vi "CRYAdd Steps.vi"() -> ()   [LabVIEW 2013]
doc: "This Example will search through the selected directory for specified files, populate the Tree control with the directory hierarchy, and then close the folder glyphs.\n This VI also demonestrates the use of the ActiveItem:RowNumber property that displays the active items row number. You could select the row number of the\n item to display its tag and cell string as well. Go to File >> VI Properties >> Documentation or Right click on the VI icon and select VI Properties. The\ncontext help window (Ctrl-h) will display detailed description of controls and indicators when you hover over them. \nInstructions:\n1. Specify the directory and the pattern to search for (i.e *.txt).\n2. Run the VI.\n3. Click on any item on the tree to display its tag and string."
uses:
  <vilib>/event_ctls.llb/eventvkey.ctl
  CRYProject/CRYProject Editor Global.vi
  CRYStepSetup/CRYStepSetup Global.vi
  CRYWindow/SubVI/CRYMain Sub Window Global.vi
  CRYMainGlobal.vi
  CRYCurveLibrary/Global/CRYCurve Library Global.vi
panel:
  in  "Option":bool
  in  "Remove":bool
  in  "StateOut":bool
  in  "Refresh":bool
  in  "UpdateAddStep":bool
  in  "stop":bool
  in  "Board Tab":enum32{"Step", "Sequence"}(tab)
  in  "Steps":string(tree)
  in  "Sequences":string(tree)
  in  "Item Remove":bool
  in  "AllChange":bool
  out "Help":string
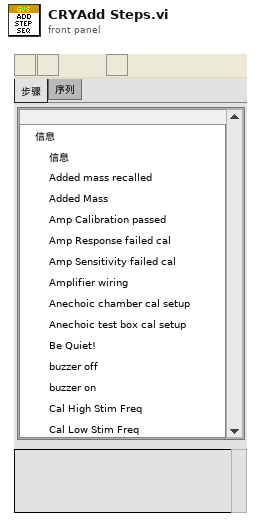
[diagram p1: front panel]
types:
  T1 = cluster{"Content":string, "Name":string, "Level":u32, "Category":string}[]
  T2 = enum16{"OK", "Yes", "YesNo", "YesNoCancel", "ReplaceAppend"}
  T3 = typedef "eventvkey.ctl" = enum16{"ASCII", "Enter", "Return", "Shift", "Ctrl", "Alt", "Cmd", "Opt", "Caps", "NumLock", "Clear", "Break", "Up", "Down", "Left", "Right", "Insert", "Delete", "Home", "End", "PageUp", "PageDown", "Escape", "Help", "Pause", "ScrollLock", "F1", "F2", "F3", "F4", "F5", "F6", "F7", "F8", "F9", "F10", "F11", "F12", "F13", "F14", "F15", "F16", "F17", "F18", "F19", "F20", "F21", "F22", "F23", "F24", "Play", "VolumeUp", "VolumeDown", "Mute", "Two Byte Char"}
  T4 = enum32{"Invalid", "Standard", "Closed", "Hidden", "Minimized", "Maximized"}
  T5 = typedef "LVPoint32TypeDef.ctl" = cluster{"Horizontal":i32, "Vertical":i32}
  T6 = cluster{"Content":string, "Name":string, "Level":u32, "Category":string}
  T7 = typedef "CRYCurveLib Info Cluster.ctl" = cluster{"GroupingState":string}
  T8 = typedef "LVRectTypeDef.ctl" = cluster{"Left":i16, "Top":i16, "Right":i16, "Bottom":i16}
  T9 = cluster{"EventName":string, "Arg1":string, "Arg1 2":string, "Numeric":dbl, "Arg1 3":string}
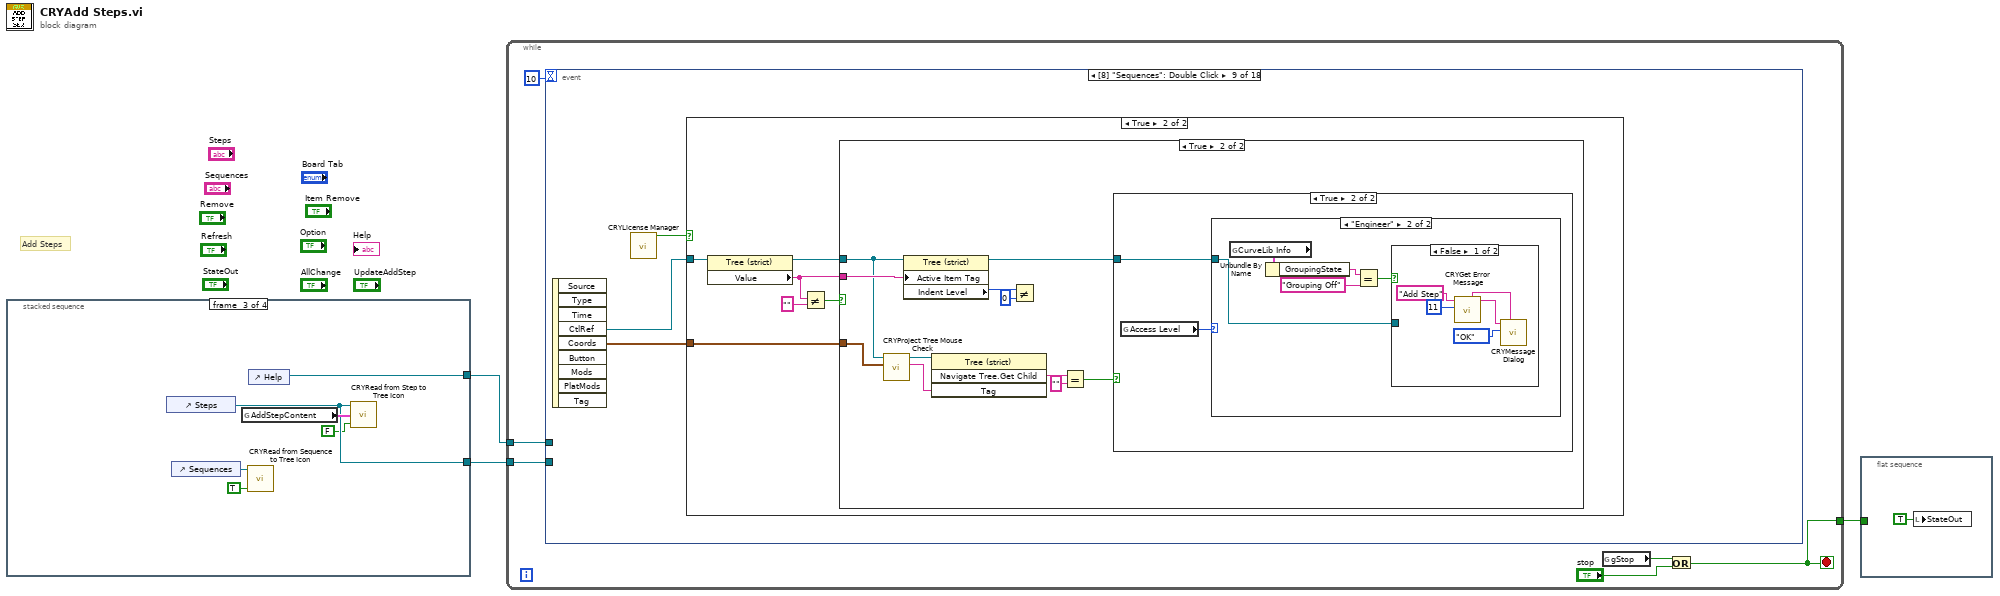
[diagram p0: block diagram]
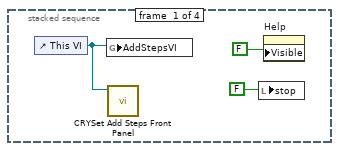
[diagram p2: hidden frame]
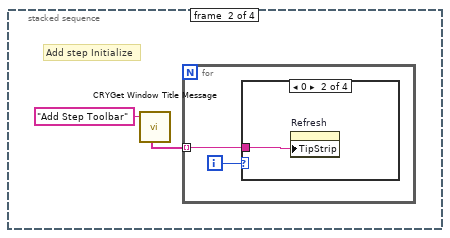
[diagram p3: hidden frame]
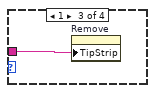
[diagram p5: hidden frame]
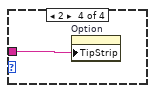
[diagram p6: hidden frame]
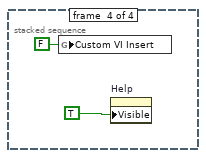
[diagram p7: hidden frame]
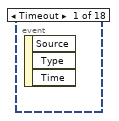
[diagram p8: hidden frame]
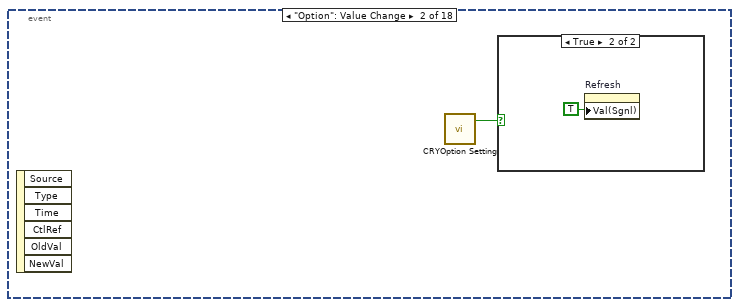
[diagram p9: hidden frame]
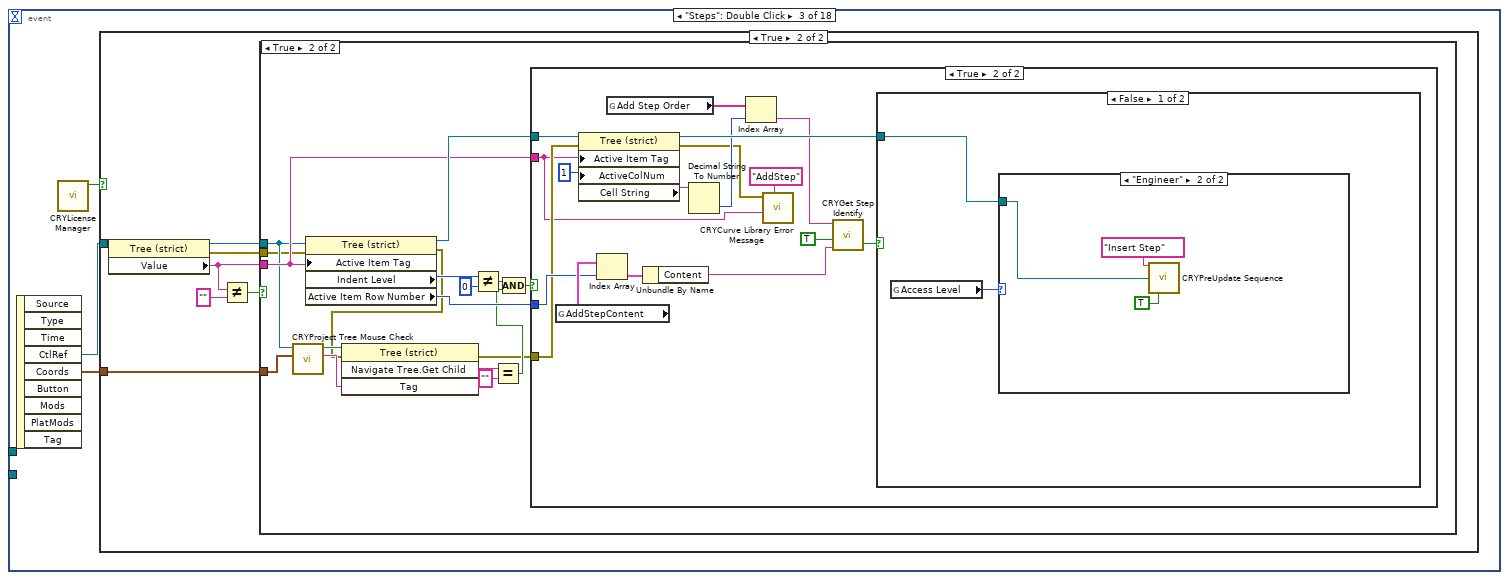
[diagram p11: hidden frame]
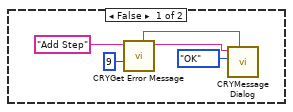
[diagram p12: hidden frame]
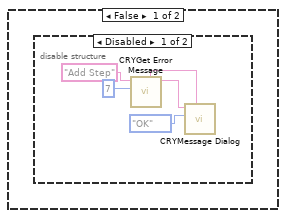
[diagram p13: hidden frame]
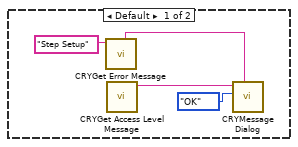
[diagram p16: hidden frame]
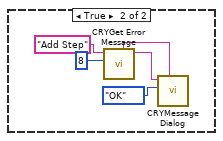
[diagram p17: hidden frame]
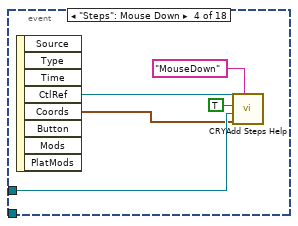
[diagram p18: hidden frame]
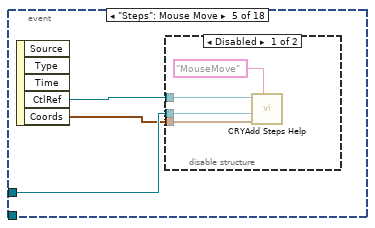
[diagram p19: hidden frame]
diagram:
  # "Add Steps"
  n1 = stacked-sequence {
    tunnel: [_ _ w19 _] -> w3
    tunnel: [_ _ w17 _] -> w2
    frame #0 {
      n2 = control-ref of="This VI"() -> (w4:refnum<vi>)
      n3 = global write "CRYProject Editor Global.vi" "AddStepsVI"(w4) -> ()
      n4 = call "CRYSet Add Steps Front Panel.vi"("Vi Ref"=w4) -> ()  [unwired: 11 in]
      n5 = local write "stop"(FALSE ("stop")) -> ()
      n6 = property on="Help" class="Str"("Visible"=FALSE) -> ()  [unwired: 2 in, 2 out]
    }
    frame #1 {
      # "Add step Initialize"
      n7 = call "CRYGet Window Title Message.vi"("Kind"="Add Step Toolbar") -> ("Tip Strip"=w8:string[])  [unwired: 5 in, 5 out]
      n8 = for {
        tunnel: w8 -> [w9] mode=indexing
        i -> [w10]
        n9 = case shown="0" w10 {
          tunnel: w9 -> [_ w11 w12 w13]
          frame Default {
          }
          frame 0 {
            n10 = property on="Refresh" class="Bool (strict)"("TipStrip"=w11) -> ()  [unwired: 2 in, 2 out]
          }
          frame 1 {
            n11 = property on="Remove" class="Bool (strict)"("TipStrip"=w12) -> ()  [unwired: 2 in, 2 out]
          }
          frame 2 {
            n12 = property on="Option" class="Bool (strict)"("TipStrip"=w13) -> ()  [unwired: 2 in, 2 out]
          }
        }
      }
    }
    frame #2 {
      n13 = control-ref of="Steps"() -> (w17:refnum<vi>)
      n14 = control-ref of="Sequences"() -> (w15:refnum<vi>)
      n15 = global read "CRYProject Editor Global.vi" "AddStepContent"() -> (w18:T1)
      n16 = call "CRYRead from Sequence to Tree Icon.vi"("Is Refresh?"=TRUE, "StepsRef in"=w15) -> ()  [unwired: 8 in, 2 out]
      n17 = control-ref of="Help"() -> (w19:refnum<vi>)
      n18 = call "CRYRead from Step to Tree Icon.vi"("Is Refresh?"=FALSE ("Type In"), "StepContentIn"=w18, "StepsRef in"=w17) -> ()  [unwired: 3 out]
    }
    frame #3 {
      n19 = global write "CRYStepSetup Global.vi" "Custom VI Insert"(FALSE ("Custom VI Insert")) -> ()
      n20 = property on="Help" class="Str"("Visible"=TRUE) -> ()  [unwired: 2 in, 2 out]
    }
  }
  n21 = while {
    tunnel: w3 -> [w26]
    tunnel: w2 -> [w25]
    tunnel: [w22] -> w1
    stop <- w22 stop-if-true
    n22 = event shown="[8] \"Sequences\": Double Click" {
      selector: _ -> [_ _ _ _ _ _ _ _ _ _ _ _ _ _ _ _ _ _]
      dyn-events: _ -> [_ _ _ _ _ _ _ _ _ _ _ _ _ _ _ _ _ _]
      timeout: 10 -> [_ _ _ _ _ _ _ _ _ _ _ _ _ _ _ _ _ _]
      tunnel: w26 -> [_ _ _ w101 w104 w113 _ _ _ _ _ _ _ _ _ _ _ _]
      tunnel: w25 -> [_ _ _ _ _ _ _ _ _ _ _ _ _ _ _ _ _ w260]
      event Timeout {
        n23 = event-data() -> ()  [unwired: 4 out]
      }
      event "Option": Value Change {
        n24 = event-data() -> ()  [unwired: 7 out]
        n25 = call "CRYOption Setting.vi"() -> ("OK Flag"=w28:bool)  [unwired: 9 in, 2 out]
        n26 = case shown="True" w28 {
          frame False {
          }
          frame True {
            n27 = property on="Refresh" class="Bool (strict)"("Val(Sgnl)"=TRUE ("Value (Signaling)")) -> ()  [unwired: 2 in, 2 out]
          }
        }
      }
      event "Steps": Double Click {
        n28 = event-data() -> ("CtlRef"=w32:refnum<vi>, "Coords"=w31:T5)  [unwired: 8 out]
        n29 = call "CRYLicense Manager.vi"() -> ("Test Result"=w30:bool)  [unwired: 10 in, 1 out]
        n30 = case shown="True" w30 {
          tunnel: w32 -> [_ w44]
          tunnel: w31 -> [_ w39]
          frame False {
            n31 = call "CRYGet Error Message.vi"("Error No"=9, "Kind"="Add Step") -> ("Message"=w33:string, "Window Title"=w37:string)  [unwired: 4 in, 4 out]
            n32 = call "CRYMessage Dialog.vi"("Window Title"=w37, "YesNoCancel"=T2."OK", "Message Content"=w33) -> ()  [unwired: 7 in, 2 out]
          }
          frame True {
            n33 = property class="Tree (strict)"(reference=w44) -> (reference out=w43:refnum<vi>, error out=w38:errorcluster, "Value"=w42:string)  [unwired: 1 in]
            n34 = Not Equal?(x=w42, y="") -> (x != y?=w40:bool)
            n35 = case shown="True" w40 {
              tunnel: w43 -> [_ w56]
              tunnel: w42 -> [_ w61]
              tunnel: w39 -> [_ w55]
              tunnel: w38 -> [_ w52]
              frame False {
                n36 = disable-structure shown="Disabled" {
                  frame Disabled {
                    n37 = call "CRYGet Error Message.vi"("Error No"=7, "Kind"="Add Step") -> ("Message"=w48:string, "Window Title"=w47:string)  [unwired: 4 in, 4 out]
                    n38 = call "CRYMessage Dialog.vi"("Window Title"=w47, "YesNoCancel"=T2."OK", "Message Content"=w48) -> ()  [unwired: 7 in, 2 out]
                  }
                  frame Enabled {
                  }
                }
              }
              frame True {
                n39 = call "CRYProject Tree Mouse Check.vi"("Coords In"=w55, "Tree Reference In"=w56) -> ("Clicked String Out"=w57:string, "Tree Reference Out"=w58:refnum<vi>)  [unwired: 8 in]
                n40 = property class="Tree (strict)"(reference=w56, error in=w52, "Active Item Tag"=w61) -> (reference out=w66:refnum<vi>, error out=w51:errorcluster, "Indent Level"=w65:i32, "Active Item Row Number"=w64:i32)
                n41 = invoke class="Tree (strict)" method="Navigate Tree.Get Child"(reference=w58, error in=w51, "Tag"=w57) -> (error out=w50:errorcluster, "Navigate Tree:Get Child"=w59:string)  [unwired: 1 in, 2 out]
                n42 = Not Equal?(x=w65, y=0) -> (x != y?=w62:bool)
                n43 = Equal?(x=w59, y="") -> (x = y?=w53:bool)
                n44 = Compound Arithmetic op=AND(w62, w53) -> (w54:bool)
                n45 = case shown="True" w54 {
                  tunnel: w64 -> [_ w78]
                  tunnel: w61 -> [_ w67]
                  tunnel: w66 -> [_ w77]
                  tunnel: w50 -> [_ w70]
                  frame False {
                  }
                  frame True {
                    n46 = global read "CRYProject Editor Global.vi" "AddStepContent"() -> (w80:T1)
                    n47 = property class="Tree (strict)"(reference=w77, error in=w70, "Active Item Tag"=w67, "ActiveColNum"=1 ("Active Cell:Active Column Number")) -> (reference out=w74:refnum<vi>, error out=w69:errorcluster, "Cell String"=w75:string)
                    n48 = Index Array(array=w80, index=w78) -> (element=w81:T6)
                    n49 = global read "CRYMainGlobal.vi" "Add Step Order"() -> (w73:string[])
                    n50 = Unbundle By Name(w81) -> ("Content"=w82:string)
                    n51 = Decimal String To Number(string=w75) -> (number=w72:i32)  [unwired: 2 in, 1 out]
                    n52 = Index Array(array=w73, index=w72) -> (element=w71:string)
                    n53 = call "CRYCurve Library Error Message.vi"("sAction"="AddStep", "sData"=w67, "error IO"=w69) -> ()  [unwired: 9 in]
                    n54 = call "CRYGet Step Identify.vi"("Unflatten Seq-step setup"=w82, "Help?"=TRUE, "Category Name In"=w71) -> ("Error?"=w79:bool)  [unwired: 1 in, 7 out]
                    n55 = case shown="False" w79 {
                      tunnel: w74 -> [w84 _]
                      frame False {
                        n56 = global read "CRYMainGlobal.vi" "Access Level"() -> (w85:enum16{"Engineer", "Technician", "Operator"})
                        n57 = case shown="\"Engineer\"" w85 {
                          tunnel: w84 -> [_ w92]
                          frame Default {
                            n58 = call "CRYGet Error Message.vi"("Kind"="Step Setup") -> ("Window Title"=w87:string)  [unwired: 5 in, 5 out]
                            n59 = call "CRYGet Access Level Message.vi"() -> ("Multibyte string"=w89:string)  [unwired: 11 in]
                            n60 = call "CRYMessage Dialog.vi"("Window Title"=w87, "YesNoCancel"=T2."OK", "Message Content"=w89) -> ()  [unwired: 7 in, 2 out]
                          }
                          frame "Engineer" {
                            n61 = call "CRYPreUpdate Sequence.vi"("EventName"="Insert Step" ("Name"), "AddSteps"=w92, "AllChangeFlg"=TRUE) -> ()  [unwired: 13 in]
                          }
                        }
                      }
                      frame True {
                        n62 = call "CRYGet Error Message.vi"("Error No"=8, "Kind"="Add Step") -> ("Message"=w96:string, "Window Title"=w95:string)  [unwired: 4 in, 4 out]
                        n63 = call "CRYMessage Dialog.vi"("Window Title"=w95, "YesNoCancel"=T2."OK", "Message Content"=w96) -> ()  [unwired: 7 in, 2 out]
                      }
                    }
                  }
                }
              }
            }
          }
        }
      }
      event "Steps": Mouse Down {
        n64 = event-data() -> ("CtlRef"=w102:refnum<vi>, "Coords"=w100:T5)  [unwired: 7 out]
        n65 = call "CRYAdd Steps Help.vi"("Option"="MouseDown", "Coords"=w100, "Help"=w101, "Help?"=TRUE, "AddSteps"=w102) -> ()  [unwired: 7 out]
      }
      event "Steps": Mouse Move {
        n66 = event-data() -> ("CtlRef"=w105:refnum<vi>, "Coords"=w103:T5)  [unwired: 4 out]
        n67 = disable-structure shown="Disabled" {
          disable-tunnel: w105 -> [w109 _]
          disable-tunnel: w104 -> [w108 _]
          disable-tunnel: w103 -> [w107 _]
          frame Disabled {
            n68 = call "CRYAdd Steps Help.vi"("Option"="MouseMove", "Coords"=w107, "Help"=w108, "AddSteps"=w109) -> ()  [unwired: 1 in, 7 out]
          }
          frame Enabled {
          }
        }
      }
      event "Steps": Key Down {
        n69 = event-data() -> ("CtlRef"=w115:refnum<vi>, "VKey"=w112:T3)  [unwired: 9 out]
        n70 = call "CRYAdd Steps Help.vi"("Option"="KeyDown", "Help"=w113, "Help?"=TRUE, "AddSteps"=w115) -> ()  [unwired: 1 in, 7 out]
        n71 = Equal?(x=w112, y=eventvkey."Delete") -> (x = y?=w110:bool)
        n72 = case shown="True" w110 {
          frame False {
          }
          frame True {
            n73 = property on="Item Remove" class="Bool (strict)"("Val(Sgnl)"=TRUE ("Value (Signaling)")) -> ()  [unwired: 2 in, 2 out]
          }
        }
      }
      event "Steps": Shortcut Menu Activation? {
        n74 = event-data() -> ("CtlRef"=w119:refnum<vi>, "MenuRef"=w120:refnum<k9>, "Coords"=w118:T5)  [unwired: 5 out]
        n75 = call "CRYGet Tree Click State.vi"("Coords"=w118, "Tree Ref In"=w119) -> ("In Bounds?"=w123:bool, "Tag"=w121:string)  [unwired: 8 out]
        n76 = Not Equal?(x=w121, y="") -> (x != y?=w124:bool)
        n77 = Compound Arithmetic op=AND(w124, w123) -> (w122:bool)
        n78 = case shown="True" w122 {
          tunnel: w120 -> [_ w128]
          tunnel: w119 -> [_ w127]
          tunnel: w121 -> [_ w126]
          frame False {
          }
          frame True {
            n79 = call "CRYAddStep Popup Menu.vi"("Tag"=w126, "Tree Reference In"=w127, "Menu Ref In"=w128) -> ()  [unwired: 8 in, 1 out]
          }
        }
        n80 = event-data() -> ()  [unwired: 2 in, 1 out]
      }
      event "Steps": Shortcut Menu Selection (User) {
        n81 = event-data() -> ("ItemTag"=w129:string)  [unwired: 8 out]
        n82 = case shown="\"AD_NEW\"" w129 {
          frame Default {
          }
          frame "AD_NEW" {
            n83 = call "CRYGet Message VI Name.vi"() -> ("Return Flag"=w131:bool, "VI Name Out"=w130:string)  [unwired: 10 in]
            n84 = case shown="True" w131 {
              tunnel: w130 -> [_ w132]
              frame False {
              }
              frame True {
                n85 = call <vilib>:"Space Constant.vi"() -> ("String"=w137:string)
                n86 = call "CRYGet Custom VIs.vi"("Category"="Custom") -> ("Custom VI Editor Names"=w135:string[])  [unwired: 10 in]
                n87 = Concatenate Strings(w132, w137, "Editor.vi" ("string")) -> (w133:string)
                n88 = Search 1D Array(1D array=w135, element=w133) -> (index of element=w134:i32)  [unwired: 1 in]
                n89 = case shown="0, Default" w134 {
                  tunnel: w133 -> [w142 _]
                  tunnel: w132 -> [w141 _]
                  frame 0, Default {
                    n90 = flat-sequence {
                      tunnel: w141 -> [w144]
                      tunnel: w142 -> [w145]
                      tunnel: [w145] -> w140
                      tunnel: [w144] -> w139
                      tunnel: w140 -> [w150]
                      tunnel: w139 -> [w146]
                      frame #0 {
                        n91 = global write "CRYStepSetup Global.vi" "Custom VI Insert"(TRUE ("Custom VI Insert")) -> ()
                      }
                      frame #1 {
                        n92 = global read "CRYMainGlobal.vi" "Custom VIs path"() -> (w151:path)
                        n93 = Build Path(base path=w151, name or relative path=w150) -> (appended path=w149:path)
                        n94 = Open VI Reference(vi path=w149) -> (vi reference=w148:refnum<vi>, error out=w147:errorcluster)  [unwired: 5 in]
                        n95 = invoke class="VI" method="Run VI"(reference=w148, error in=w147, "Wait until done"=FALSE ("Wait Until Done")) -> (reference out=w153:refnum<vi>, error out=w152:errorcluster)  [unwired: 2 in, 3 out]
                        n96 = property class="VI"(reference=w153, error in=w152, "Front Panel.Title"=w146) -> (reference out=w155:refnum<vi>, error out=w154:errorcluster)
                        n97 = property class="VI"(reference=w155, error in=w154, "Front Panel Window:Open"=TRUE ("Front Panel.Open")) -> ()  [unwired: 2 out]
                      }
                    }
                  }
                  frame -1 {
                    n98 = call "CRYGet Error Message.vi"("Error No"=10, "Kind"="Add Step") -> ("Message"=w161:string, "Window Title"=w162:string)  [unwired: 4 in, 4 out]
                    n99 = call "CRYMessage Dialog.vi"("Window Title"=w162, "YesNoCancel"=T2."OK", "Message Content"=w161) -> ()  [unwired: 7 in, 2 out]
                  }
                }
              }
            }
          }
        }
      }
      event "Sequences": Double Click {
        n100 = event-data() -> ("CtlRef"=w165:refnum<vi>, "Coords"=w164:T5)  [unwired: 8 out]
        n101 = call "CRYLicense Manager.vi"() -> ("Test Result"=w163:bool)  [unwired: 10 in, 1 out]
        n102 = case shown="True" w163 {
          tunnel: w165 -> [_ w175]
          tunnel: w164 -> [_ w171]
          frame False {
            n103 = call "CRYGet Error Message.vi"("Error No"=9, "Kind"="Add Step") -> ("Message"=w166:string, "Window Title"=w170:string)  [unwired: 4 in, 4 out]
            n104 = call "CRYMessage Dialog.vi"("Window Title"=w170, "YesNoCancel"=T2."OK", "Message Content"=w166) -> ()  [unwired: 7 in, 2 out]
          }
          frame True {
            n105 = property class="Tree (strict)"(reference=w175) -> (reference out=w172:refnum<vi>, "Value"=w173:string)  [unwired: 1 in, 1 out]
            n106 = Not Equal?(x=w173, y="") -> (x != y?=w174:bool)
            n107 = case shown="True" w174 {
              tunnel: w173 -> [_ w189]
              tunnel: w172 -> [_ w184]
              tunnel: w171 -> [_ w183]
              frame False {
                n108 = disable-structure shown="Disabled" {
                  frame Disabled {
                    n109 = call "CRYGet Error Message.vi"("Error No"=7, "Kind"="Add Step") -> ("Message"=w180:string, "Window Title"=w179:string)  [unwired: 4 in, 4 out]
                    n110 = call "CRYMessage Dialog.vi"("Window Title"=w179, "YesNoCancel"=T2."OK", "Message Content"=w180) -> ()  [unwired: 7 in, 2 out]
                  }
                  frame Enabled {
                  }
                }
              }
              frame True {
                n111 = call "CRYProject Tree Mouse Check.vi"("Coords In"=w183, "Tree Reference In"=w184) -> ("Clicked String Out"=w185:string, "Tree Reference Out"=w186:refnum<vi>)  [unwired: 8 in]
                n112 = property class="Tree (strict)"(reference=w184, "Active Item Tag"=w189) -> (reference out=w190:refnum<vi>, "Indent Level"=w192:i32)  [unwired: 1 in, 1 out]
                n113 = invoke class="Tree (strict)" method="Navigate Tree.Get Child"(reference=w186, "Tag"=w185) -> ("Navigate Tree:Get Child"=w187:string)  [unwired: 2 in, 3 out]
                n114 = Not Equal?(x=w192, y=0) -> ()  [unwired: 1 out]
                n115 = Equal?(x=w187, y="") -> (x = y?=w182:bool)
                n116 = case shown="True" w182 {
                  tunnel: w190 -> [_ w194]
                  frame False {
                  }
                  frame True {
                    n117 = global read "CRYMainGlobal.vi" "Access Level"() -> (w193:enum16{"Engineer", "Technician", "Operator"})
                    n118 = case shown="\"Engineer\"" w193 {
                      tunnel: w194 -> [_ w203]
                      frame Default {
                        n119 = call "CRYGet Error Message.vi"("Kind"="Step Setup") -> ("Window Title"=w197:string)  [unwired: 5 in, 5 out]
                        n120 = call "CRYGet Access Level Message.vi"() -> ("Multibyte string"=w195:string)  [unwired: 11 in]
                        n121 = call "CRYMessage Dialog.vi"("Window Title"=w197, "YesNoCancel"=T2."OK", "Message Content"=w195) -> ()  [unwired: 7 in, 2 out]
                      }
                      frame "Engineer" {
                        n122 = global read "CRYCurve Library Global.vi" "CurveLib Info"() -> (w202:T7)
                        n123 = Unbundle By Name(w202) -> ("GroupingState"=w201:string)
                        n124 = Equal?(x=w201, y="Grouping Off") -> (x = y?=w199:bool)
                        n125 = case shown="False" w199 {
                          tunnel: w203 -> [_ w211]
                          frame False {
                            n126 = call "CRYGet Error Message.vi"("Error No"=11, "Kind"="Add Step") -> ("Message"=w207:string, "Window Title"=w206:string)  [unwired: 4 in, 4 out]
                            n127 = call "CRYMessage Dialog.vi"("Window Title"=w206, "YesNoCancel"=T2."OK", "Message Content"=w207) -> ()  [unwired: 7 in, 2 out]
                          }
                          frame True {
                            n128 = call "CRYPreUpdate Sequence.vi"("EventName"="Insert Sequence" ("Name"), "AddSteps"=w211, "AllChangeFlg"=TRUE) -> ()  [unwired: 13 in]
                          }
                        }
                      }
                    }
                  }
                }
              }
            }
          }
        }
      }
      event "Sequences": Mouse Down {
        n129 = event-data() -> ()  [unwired: 9 out]
      }
      event "Sequences": Key Down {
        n130 = event-data() -> ("VKey"=w212:T3)  [unwired: 10 out]
        n131 = Equal?(x=w212, y=eventvkey."Delete") -> (x = y?=w213:bool)
        n132 = case shown="True" w213 {
          frame False {
          }
          frame True {
            n133 = property on="Item Remove" class="Bool (strict)"("Val(Sgnl)"=TRUE ("Value (Signaling)")) -> ()  [unwired: 2 in, 2 out]
          }
        }
      }
      event Pane Size {
        w221 = 0 ("Active Cell:Active Column Number")
        n134 = event-data() -> ("NewBnds"=w229:T8)  [unwired: 6 out]
        n135 = Unbundle By Name(w229) -> ("Right"=w227:i16, "Left"=w228:i16, "Bottom"=w226:i16, "Top"=w225:i16)
        n136 = Subtract(x=w227, y=w228) -> (x-y=w218:i16)
        n137 = Subtract(x=w226, y=w225) -> (x-y=w223:i16)
        n138 = Subtract(x=w218, y=i16 5) -> (x-y=w219:i16)
        n139 = Subtract(x=w223, y=i16 33) -> (x-y=w220:i16)
        n140 = control-ref of="Steps"() -> (w216:refnum<vi>)
        n141 = property on="Property Node" class="Tree (strict)"(reference=w216, "Width"=w218, "ActiveColNum"=w221, "Width"=w219, "Height"=w220) -> ()  [unwired: 1 in, 2 out]
        n142 = control-ref of="Sequences"() -> (w217:refnum<vi>)
        n143 = property on="Property Node" class="Tree (strict)"(reference=w217, "Width"=w218, "ActiveColNum"=w221, "Width"=w219, "Height"=w220) -> ()  [unwired: 1 in, 2 out]
      }
      event Panel Close? {
        n144 = event-data() -> ()  [unwired: 5 out]
        n145 = control-ref of="This VI"() -> (w231:refnum<vi>)
        n146 = invoke class="VI" method="FP.Open"(reference=w231, "Activate"=TRUE ("Front Panel Window:Open"), "State"=T4."Hidden") -> ()  [unwired: 2 in, 5 out]
        n147 = event-data("Discard?"=TRUE) -> ()  [unwired: 1 in, 1 out]
      }
      event "Refresh": Value Change {
        n148 = event-data() -> ()  [unwired: 7 out]
        n149 = flat-sequence {
          frame #0 {
            n150 = call "CRYStep Contents Init.vi"() -> ()  [unwired: 12 in]
          }
          frame #1 {
            n151 = control-ref of="Steps"() -> (w238:refnum<vi>)
            n152 = global read "CRYProject Editor Global.vi" "AddStepContent"() -> (w239:T1)
            n153 = call "CRYRead from Step to Tree Icon.vi"("Is Refresh?"=TRUE ("Type In"), "StepContentIn"=w239, "StepsRef in"=w238) -> ()  [unwired: 3 out]
          }
          frame #2 {
            n154 = control-ref of="Sequences"() -> (w240:refnum<vi>)
            n155 = call "CRYRead from Sequence to Tree Icon.vi"("Is Refresh?"=TRUE, "StepsRef in"=w240) -> ()  [unwired: 8 in, 2 out]
          }
          frame #3 {
            n156 = call "CRYProject Editor PIC Action End.vi"() -> ()  [unwired: 12 in]
          }
        }
        n157 = call "CRYGet Window Title Message.vi"("No"=2 ("Error No"), "Kind"="Add Step") -> ("Unicode String"=w234:string)  [unwired: 4 in, 5 out]
        n158 = call "CRYProject Editor PIC Action Start.vi"("sData"=w234) -> ()  [unwired: 11 in]
      }
      event "Remove": Value Change {
        n159 = event-data() -> ()  [unwired: 7 out]
        n160 = property on="Item Remove" class="Bool (strict)"("Val(Sgnl)"=TRUE ("Value (Signaling)")) -> ()  [unwired: 2 in, 2 out]
      }
      event "Item Remove": Value Change {
        n161 = event-data() -> ("CtlRef"=w246:refnum<vi>)  [unwired: 6 out]
        n162 = property class="Bool (strict)"(reference=w246, "Value"=FALSE) -> ()  [unwired: 1 in, 2 out]
        n163 = local read "Board Tab"() -> (w245:enum32{"Step", "Sequence"})
        n164 = case shown="\"Sequence\"" w245 {
          tunnel: ["Step Remove" ("Option") "Sequence Remove" ("Option")] -> w244
          tunnel: [w248 w250] -> w243
          frame "Step", Default {
            n165 = control-ref of="Steps"() -> (w248:refnum<vi>)
          }
          frame "Sequence" {
            n166 = control-ref of="Sequences"() -> (w250:refnum<vi>)
          }
        }
        n167 = call "CRYAdd Step Intem Remove.vi"("AddSteps"=w243, "Option"=w244) -> ()  [unwired: 10 in]
      }
      event "AllChange": Value Change {
        n168 = event-data() -> ("CtlRef"=w254:refnum<vi>)  [unwired: 6 out]
        n169 = property class="Bool (strict)"(reference=w254, "Value"=FALSE) -> ()  [unwired: 1 in, 2 out]
        n170 = global read "CRYProject Editor Global.vi" "AddStepCluster"() -> (w253:T9)
        n171 = Unbundle By Name(w253) -> ("EventName"=w252:string)
        n172 = case shown="\"UpdateAddStep\"" w252 {
          frame "False", Default {
          }
          frame "UpdateAddStep" {
            n173 = property on="Refresh" class="Bool (strict)"("Val(Sgnl)"=TRUE ("Value (Signaling)")) -> ()  [unwired: 2 in, 2 out]
          }
        }
      }
      event "UpdateAddStep": Value Change {
        n174 = event-data() -> ()  [unwired: 7 out]
        n175 = flat-sequence {
          tunnel: w260 -> [w261]
          frame #0 {
            n176 = global read "CRYProject Editor Global.vi" "AddStepCluster"() -> (w265:T9)
            n177 = Unbundle By Name(w265) -> ("Arg1"=w264:string, "Arg1 2"=w263:string, "Arg1 3"=w262:string)  [unwired: 1 out]
            n178 = call "CRYUpdate Steps.vi"("AddStepsTree"=w261, "Category Name"=w264, "Step flattened"=w262, "StepFileName"=w263) -> ()  [unwired: 8 out]
          }
          frame #1 {
            n179 = call "CRYProject Editor PIC Action End.vi"() -> ()  [unwired: 12 in]
            n180 = control-ref of="Sequences"() -> (w266:refnum<vi>)
            n181 = call "CRYRead from Sequence to Tree Icon.vi"("StepsRef in"=w266) -> ()  [unwired: 9 in, 2 out]
          }
        }
        n182 = call "CRYGet Window Title Message.vi"("No"=3 ("Error No"), "Kind"="Add Step") -> ("Unicode String"=w257:string)  [unwired: 4 in, 5 out]
        n183 = call "CRYProject Editor PIC Action Start.vi"("sData"=w257) -> ()  [unwired: 11 in]
      }
    }
    n184 = global read "CRYMain Sub Window Global.vi" "gStop"() -> (w24:bool)
    n185 = Or(x=w24, y="stop") -> (x .or. y?=w22:bool)
  }
  n186 = flat-sequence {
    tunnel: w1 -> [_]
    frame #0 {
      n187 = local write "StateOut"(TRUE ("StateOut")) -> ()
    }
  }
